vi "testNoError.vi"() -> ()   [LabVIEW 2017, in "AssertionTest.lvlib" / "ErrorMessageContainsString.lvlib"]
uses:
  ErrorMessageContainsString.lvlib
  Assertion/Assertion.lvlib
  AssertionTest.lvlib
  a9cd2165-557e-43d9-abd3-def871d88858.vi
panel:
  out "error out":errorcluster
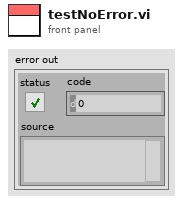
[diagram p1: front panel]
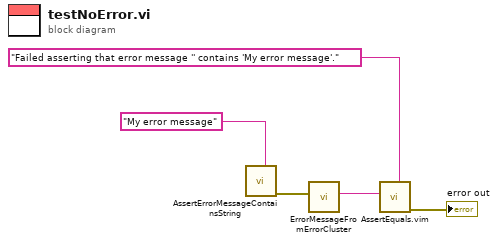
[diagram p0: block diagram]
diagram:
  n1 = call "AssertErrorMessageContainsString.vi"("Expected"="My error message") -> ("error out"=w2:errorcluster)  [unwired: 10 in]
  n2 = call "ErrorMessageFromErrorCluster.vi"("Error"=w2) -> ("Error Message"=w4:string)  [unwired: 10 in]
  n3 = call "AssertEquals.vim"("Expected"="Failed asserting that error message '' contains 'My error message'." ("Needle"), "Actual"=w4) -> ("error out"=→"error out":errorcluster)  [unwired: 9 in]
